vi "Fetch Trace (Channel Power Measurement).vi"(0 "VISA resource name":refnum<visa-resource-name>, 5 "Timeout (10000 ms)":i32=10000 format="%.0g", 11 "error in (no error)":errorcluster) -> (4 "VISA resource name out":refnum<visa-resource-name>, 6 "Initial X":dbl, 8 "X Increment":dbl, 10 "Trace Array":dbl[](array[numeric]), 15 "error out":errorcluster)   [LabVIEW 2018, in "Agilent MXA Series.lvlib"]
doc: "Fetches trace from the spectrum analyzer (Channel Power Measurement) and does not initiate data acquisition.\n\n<B>Note:</B>\n\nUse this VI only with other low-level VIs. The high-level VIs automatically incorporate this functionality. This VI does not check the instrument status."
uses:
  Agilent MXA Series.lvlib
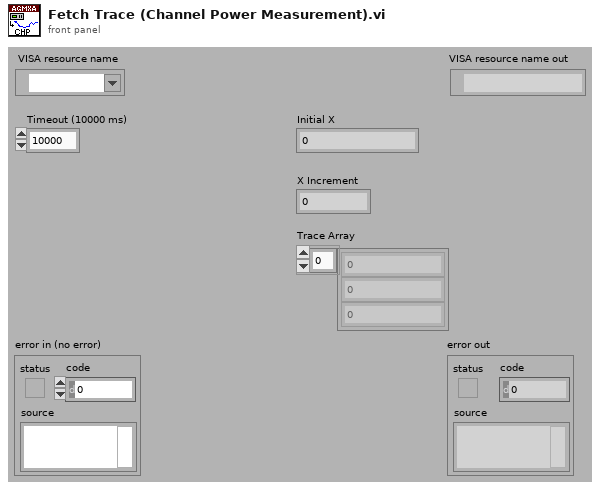
[diagram p1: front panel]
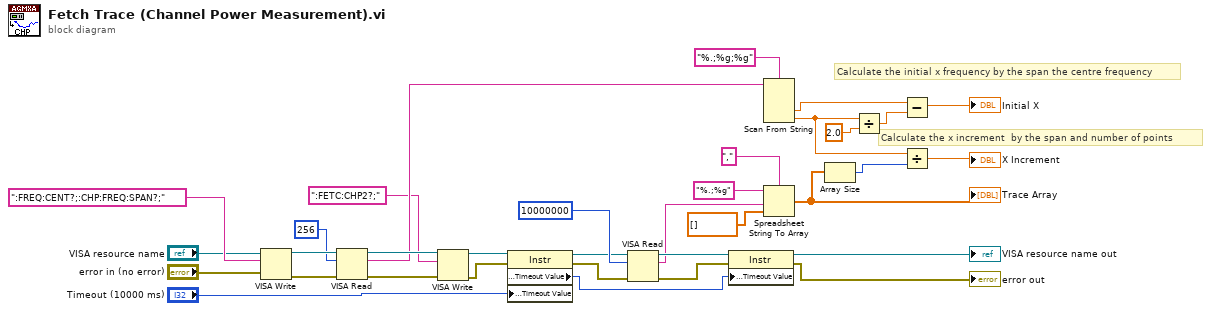
[diagram p0: block diagram]
diagram:
  # "Calculate the x increment  by the span and number of points"
  # "Calculate the initial x frequency by the span the centre frequency"
  n1 = VISA Write(VISA resource name="VISA resource name", write buffer=":FREQ:CENT?;:CHP:FREQ:SPAN?;", error in (no error)="error in (no error)") -> (VISA resource name out=w31:refnum<visa-resource-name>, error out=w30:errorcluster)  [unwired: 1 out]
  n2 = VISA Read(VISA resource name=w31, byte count=256, error in (no error)=w30) -> (VISA resource name out=w11:refnum<visa-resource-name>, read buffer=w7:string, error out=w10:errorcluster)  [unwired: 1 out]
  n3 = VISA Write(VISA resource name=w11, write buffer=":FETC:CHP2?;", error in (no error)=w10) -> (VISA resource name out=w22:refnum<visa-resource-name>, error out=w21:errorcluster)  [unwired: 1 out]
  n4 = property on="Property Node" class="Instr"(reference=w22, error in=w21, "General Settings:Timeout Value"="Timeout (10000 ms)") -> (reference out=w27:refnum<visa-resource-name>, error out=w26:errorcluster, "General Settings:Timeout Value"=w23:u32)
  n5 = VISA Read(VISA resource name=w27, byte count=10000000, error in (no error)=w26) -> (VISA resource name out=w25:refnum<visa-resource-name>, read buffer=w17:string, error out=w24:errorcluster)  [unwired: 1 out]
  n6 = property on="Property Node" class="Instr"(reference=w25, error in=w24, "General Settings:Timeout Value"=w23) -> (reference out=→"VISA resource name out":refnum<visa-resource-name>, error out=→"error out":errorcluster)
  n7 = Scan From String(format string="%.;%g;%g", input string=w7) -> (output 1=w15:dbl, output 2=w13:dbl)  [unwired: 4 in, 3 out]
  n8 = Spreadsheet String To Array(delimiter (Tab)=",", format string="%.;%g", spreadsheet string=w17, array type (2D Dbl)=dbl[] []) -> (array=w5:dbl[])
  "Trace Array" <- w5
  n9 = Array Size(array=w5) -> (size(s)=w12:i32)
  n10 = Divide(x=w13, y=2.0) -> (x/y=w14:dbl)
  n11 = Subtract(x=w15, y=w14) -> (x-y=→"Initial X":dbl)
  n12 = Divide(x=w13, y=w12) -> (x/y=→"X Increment":dbl)
